vi "finishPassTo2ndStrikerPlay.vi"(8 "error in (no error)":errorcluster, 10 "Game":refnum<class "Game.lvclass">, 11 "PassTo2ndStriker in":refnum<class "PassTo2ndStriker.lvclass">) -> (0 "error out":errorcluster, 1 "OffensiveTeam":refnum<class "Ally.lvclass">, 2 "finishPassTo2ndStriker?":bool, 3 "PassTo2ndStriker out":refnum<class "PassTo2ndStriker.lvclass">)   [LabVIEW 2020, in "PassTo2ndStriker.lvclass"]
uses:
  PassTo2ndStriker.lvclass
  Game_class/Game.lvclass
  Ally_class/Ally.lvclass
  Referee_class/command_interpreted.ctl
  Utilities_class/Utilities.lvclass
  Game_class/Game.lvclass/Game.ctl
  Referee_class/Referee.lvclass/Referee.ctl
  Events_class/Events.lvclass/Events.ctl
  Object_class/Object.lvclass/Object.ctl
  Ball_class/Ball.lvclass/Ball.ctl
  Team_class/Team.lvclass/Team.ctl
  Ally_class/Ally.lvclass/Ally.ctl
  Ally_class/Read PreparePassPlaysEnum.vi
  Ally_class/Write PreparePassPlaysEnum.vi
  Game_class/Read EventsRef.vi
  Game_class/Read BallRef.vi
  Game_class/Read OffensiveTeam.vi
  Team_class/Read RobotRef.vi
  Object_class/Read x.vi
  Object_class/Read y.vi
  Ball_class/Read z.vi
  Events_class/Read touch.vi
  Events_class/Read enemy_ball_possesion.vi
  Events_class/Read id_touch.vi
  Events_class/Read ball_out.vi
  Game_class/Read Referee.vi
  Referee_class/Read command_interpreted.vi
  Ball_class/Ball.lvclass
  Referee_class/Referee.lvclass
  Events_class/Events.lvclass
  Robot_class/Robot.lvclass
  Play_class/Play.lvclass
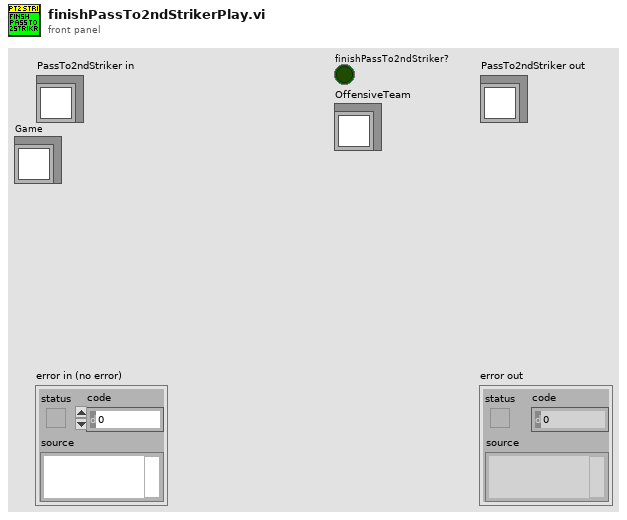
[diagram p1: front panel]
types:
  T1 = typedef "command_interpreted.ctl" = enum16{"Goal Ally", "Goal Enemy", "Ball Placement Enemy", "Ball Placement Ally", "Normal Half Time", "Extra Time  Break", "Extra Half Time", "None", "Post Game", "PKA Normal Start", "Prepare Kickoff Ally", "PKE Normal Start", "Prepare Kickoff Enemy", "Force Start", "Halt", "Timeout", "Prepare Penalty Ally", "Prepare Penalty Enemy", "PPA NormalStart", "PPE Normal Start", "Indirect Free Ally", "Direct Free Enemy", "Direct Free Ally", "Indirect Free Enemy", "Stop"}
  T2 = typedef "OffensivePlay.ctl" = enum16{"PrepareFourthPass", "KeeperPassToStriker", "PrepareKeeperPass", "ACBPass", "ABCPass", "PrepareTriplePass", "TableWithStriker", "TableWith2ndStrikerPlay", "PrepareDoublePass", "PrepareRollToPass", "SimplePass", "PreparePass", "PassToStriker", "BallOutOfField", "PassTo2ndStriker", "StopOffensive", "Prepare Penalty Enemy", "EnemyPossessionAtEnemyField", "EnemyPossesionAtOurField", "TestPlay", "PreparePenaltyAlly", "KickPenaltyAlly", "PrepareKickoffAlly", "PrepareKickoffEnemy", "IndirectEnemy", "DirectEnemy", "PreparePassInGame1", "NormalGame", "DirectKick", "Pass", "Halt", "Timeout", "PassPlay", "PenaltyEnemy"}
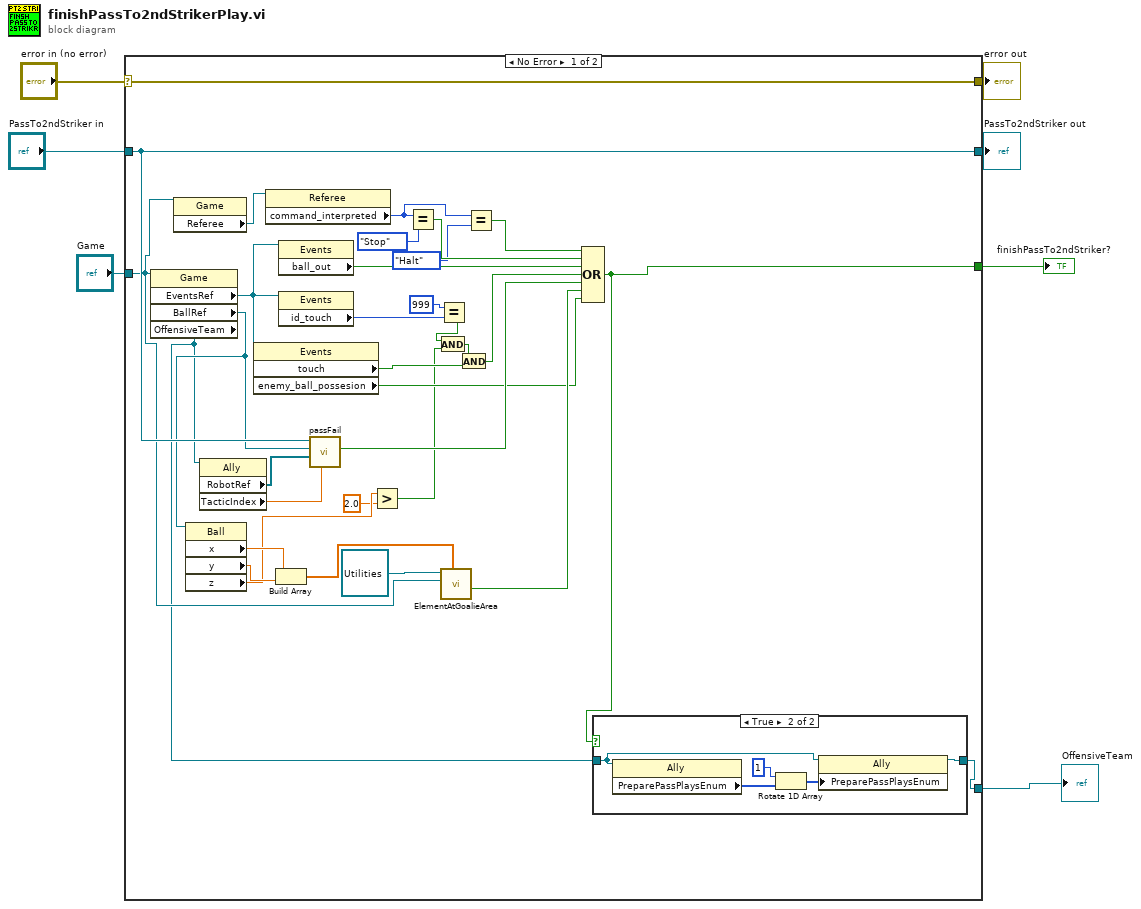
[diagram p0: block diagram]
diagram:
  n1 = case shown="No Error" "error in (no error)" {
    selector: "error in (no error)" -> [w40 w48]
    tunnel: [w40 w48] -> w6
    tunnel: [w19 w47] -> w4
    tunnel: "PassTo2ndStriker in" -> [w19 w47]
    tunnel: [w8 _] -> w3
    tunnel: "Game" -> [w18 _]
    tunnel: [w10 _] -> w1
    frame No Error {
      n2 = property class="Game"(reference=w18) -> ("EventsRef"=w39:refnum<class "Events.lvclass">, "BallRef"=w17:refnum<class "Ball.lvclass">, "OffensiveTeam"=w9:refnum<class "Ally.lvclass">)  [unwired: 1 in, 2 out]
      n3 = property class="Game"(reference=w18) -> ("Referee"=w34:refnum<class "Referee.lvclass">)  [unwired: 1 in, 2 out]
      n4 = property class="Ball"(reference=w17) -> ("x"=w23:dbl, "y"=w22:dbl, "z"=w15:dbl)  [unwired: 1 in, 2 out]
      n5 = property class="Ally"(reference=w9) -> ("RobotRef"=w27:refnum<class "Robot.lvclass">[], "TacticIndex"=w25:dbl)  [unwired: 1 in, 2 out]
      n6 = property class="Events"(reference=w39) -> ("touch"=w33:bool, "enemy_ball_possesion"=w16:bool)  [unwired: 1 in, 2 out]
      n7 = property class="Referee"(reference=w34) -> ("command_interpreted"=w30:T1)  [unwired: 1 in, 2 out]
      n8 = Build Array(w23, w22) -> (w21:dbl[])
      n9 = property class="Events"(reference=w39) -> ("ball_out"=w36:bool)  [unwired: 1 in, 2 out]
      n10 = property class="Events"(reference=w39) -> ("id_touch"=w37:i32)  [unwired: 1 in, 2 out]
      n11 = call "passFail.vi"("TacticIndex"=w25, "Offensive Robots"=w27, "Ball"=w17, "Play in"=w19) -> ("PassFail?"=w26:bool)  [unwired: 5 in, 2 out]
      n12 = Greater?(x=w15, y=2.0) -> (0:w12:bool)
      n13 = Equal?(x=w30, y=command_interpreted."Stop" ("command_interpreted")) -> (x = y?=w31:bool)
      n14 = Equal?(x=999 ("id_touch"), y=w37) -> (x = y?=w13:bool)
      n15 = And(x=w13, y=w12) -> (x .and. y?=w11:bool)
      n16 = call-dynamic "ElementAtGoalieArea.vi"("Elemento pos."=w21, "Game"=w18, "Utilities in"=refnum<class "Utilities.lvclass"> refnum) -> ("Element at our goalkeeper area ?"=w20:bool)  [unwired: 5 in, 3 out]
      n17 = And(x=w11, y=w33) -> (x .and. y?=w35:bool)
      n18 = Equal?(x=w30, y=command_interpreted."Halt" ("command_interpreted")) -> (x = y?=w28:bool)
      n19 = Compound Arithmetic op=OR(w28, w31, w36, w35, w26, w20, w16) -> (w8:bool)
      n20 = case shown="True" w8 {
        tunnel: w9 -> [w41 w43]
        tunnel: [w41 w42] -> w10
        frame False {
        }
        frame True {
          n21 = property class="Ally"(reference=w43) -> ("PreparePassPlaysEnum"=w44:T2[])  [unwired: 1 in, 2 out]
          n22 = Rotate 1D Array(1:w44, 2:1 ("n")) -> (0:w45:T2[])
          n23 = property class="Ally"(reference=w43, "PreparePassPlaysEnum"=w45) -> (reference out=w42:refnum<class "Ally.lvclass">)  [unwired: 1 in, 1 out]
        }
      }
    }
    frame Error {
    }
  }
  "error out" <- w6
  "PassTo2ndStriker out" <- w4
  "finishPassTo2ndStriker?" <- w3
  "OffensiveTeam" <- w1
